vi "camera_acquisition_cooper.vi"(9 "Pixel Clock":dbl, 10 "Frame Rate":dbl) -> ()   [LabVIEW 2016]
uses:
  C:/Users/RegA/Box/bokor/cooper/32_bit/Library_X86/Thorlabs.TSI.ImageDataInterfaces.dll
  C:/Users/RegA/Box/bokor/cooper/32_bit/Library_X86/Thorlabs.TSI.TLCameraInterfaces.dll
  <vilib>/Analysis/NI_AALBase.lvlib
  C:/Users/RegA/Box/bokor/cooper/32_bit/Library_X86/Thorlabs.TSI.TLCamera.dll
  <vilib>/Analysis/baseanly.llb/A x Vector.vi
  <vilib>/Utility/file.llb/Write Delimited Spreadsheet (string).vi
  <vilib>/Utility/file.llb/Write Delimited Spreadsheet (DBL).vi
panel:
  in  "Subtract\nBackground":bool
  in  "Calibrate\nBackground":bool
  out "Background":u8[][](graph)
  in  "Stop Recording":bool
  out "Recording In\nProgress":bool
  in  "File Name (3):":string="GdFeCo202_"
  in  "Save at (3):":path=path "C:/Users/Bokor Group/Google Drive/MOKE_Microscopy/11_2016/Nov14"
  in  "Start Recording":bool
  out "Recording\nFrames":dbl
  out "Recording\nLength":dbl
  out "Scan in\nProgress":bool
  in  "Amplifier\nGPIB":refnum<visa-resource-name>="GPIB0::8::INSTR"
  in  "Enable Manual Control":bool
  in  "File Name (2):":string="GdFeCo202_"
  in  "Save at (2):":path=path "C:/Users/Bokor Group/Google Drive/MOKE_Microscopy/11_2016/Nov14"
  in  "Kepco\nGPIB":refnum<visa-resource-name>="GPIB0::8::INSTR"
  in  "Number\nOf Loops":dbl=1.0
  in  "Set I\nDelay":dbl=0.5
  in  "Stop\nScan":bool
  out "Hysteresis\nGraph":cluster{dbl[], dbl[]}(graph)={[0.0, 0.05, 0.1, 0.15000000000000002, 0.2, 0.25, 0.3, 0.0], [5.96051e-08, 8.56821e-08, 5.21543e-08, 2.98025e-08, 6.33304e-08, 7.0781e-08, 9.31327e-08, 1.00583e-07]}
  in  "Step (A)":dbl=0.05 format="%.5f"
  in  "-Imax (A)":dbl=-0.5
  in  "Imax (A)":dbl=0.5
  in  "Kepco Control Value":dbl(knob) min=-3.0 max=3.0 step=0.01 scale=-0.5..0.5 scale format="%#_3g"
  in  "Start\nScan":bool
  in  "Save\nScan":bool
  in  "File Name (1):":string="GdFeCo202_"
  in  "Save At (1):":path=path "C:/Users/Bokor Group/Google Drive/MOKE_Microscopy/11_2016/Nov14"
  in  "Take Pic":bool
  out "Pic Taken":u8[][](graph)
  in  "Exposure (ms)":u32=100
  in  "Intensity\nRange":cluster{dbl, dbl}(slide)={56.92307692307693, 40.0} scale=40.0..160.0
  out "Average":dbl=48.534001159667945
  out "Video":u8[][](graph)
  in  "Maximum\nIntensity":bool
  in  "stop":bool
  # "Save Pic"
  # "Save Video"
  # "Stop Button"
  # "Save Hysteresis Scan"
  # "Control Kepco"
  # "Background"
  # "A"
  # "Camera Image"
  # "Run Hysteresis Loop"
  # "Kepco GPIB"
  # "Unused"
  # "Amplifier GPIB"
  # "Unused"
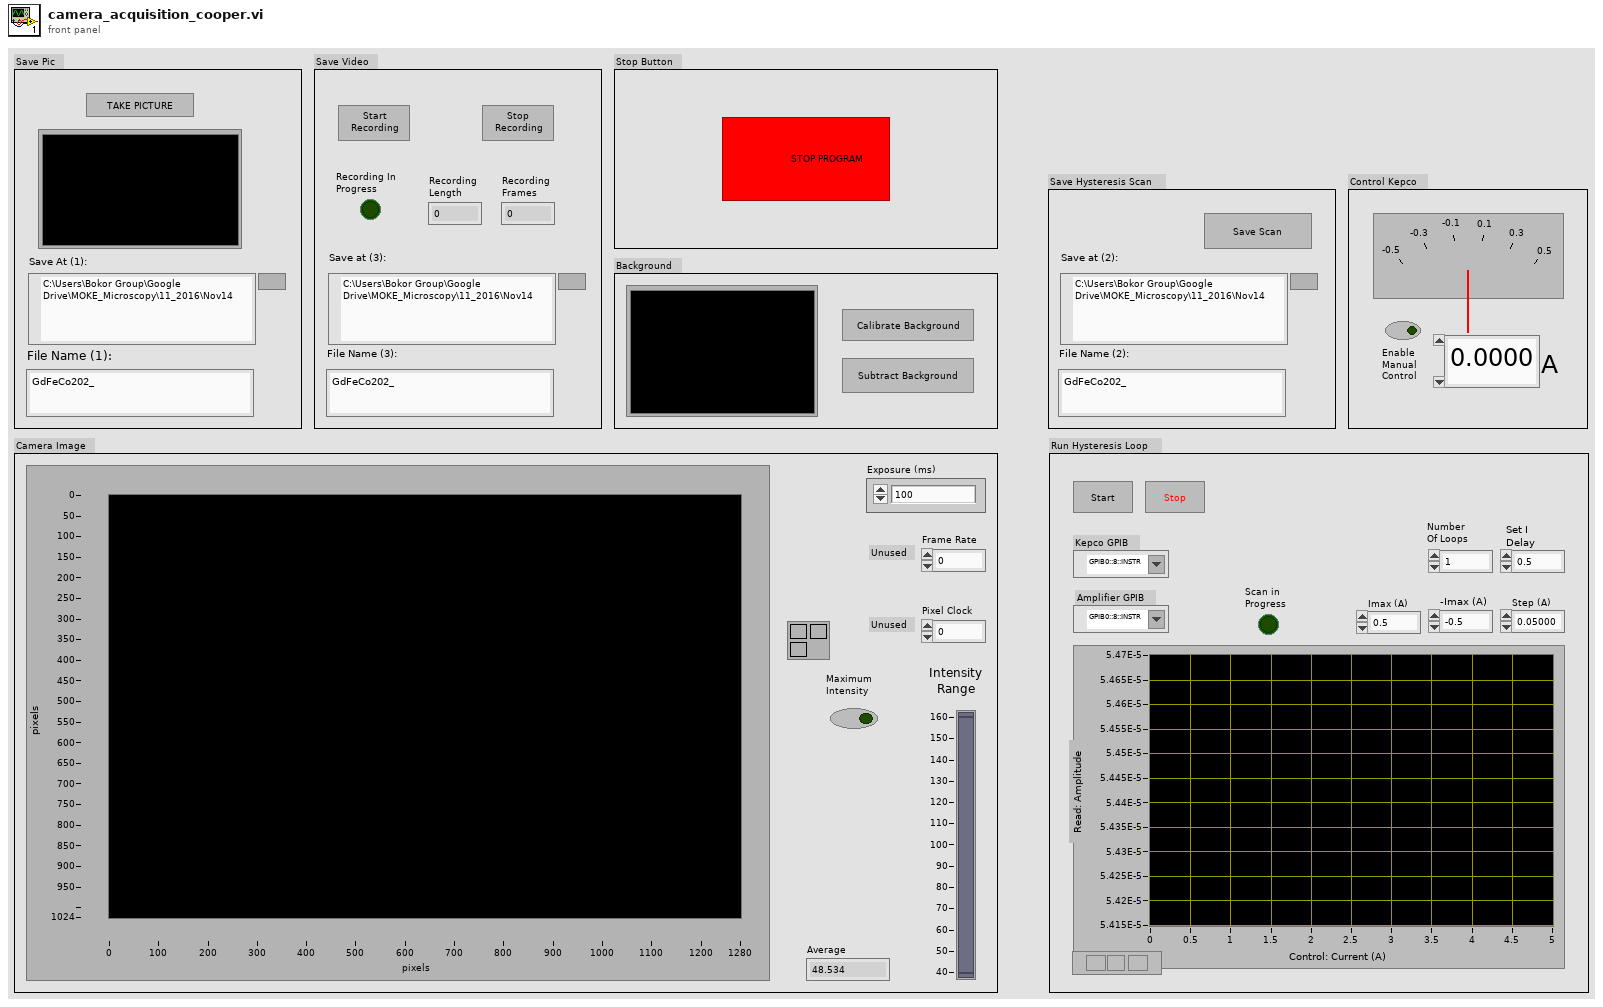
[diagram p1: front panel]
types:
  T1 = typedef "IMAQ Image.ctl" = refnum<image>
  T2 = typedef "AviRefnum.ctl" = refnum<k1>
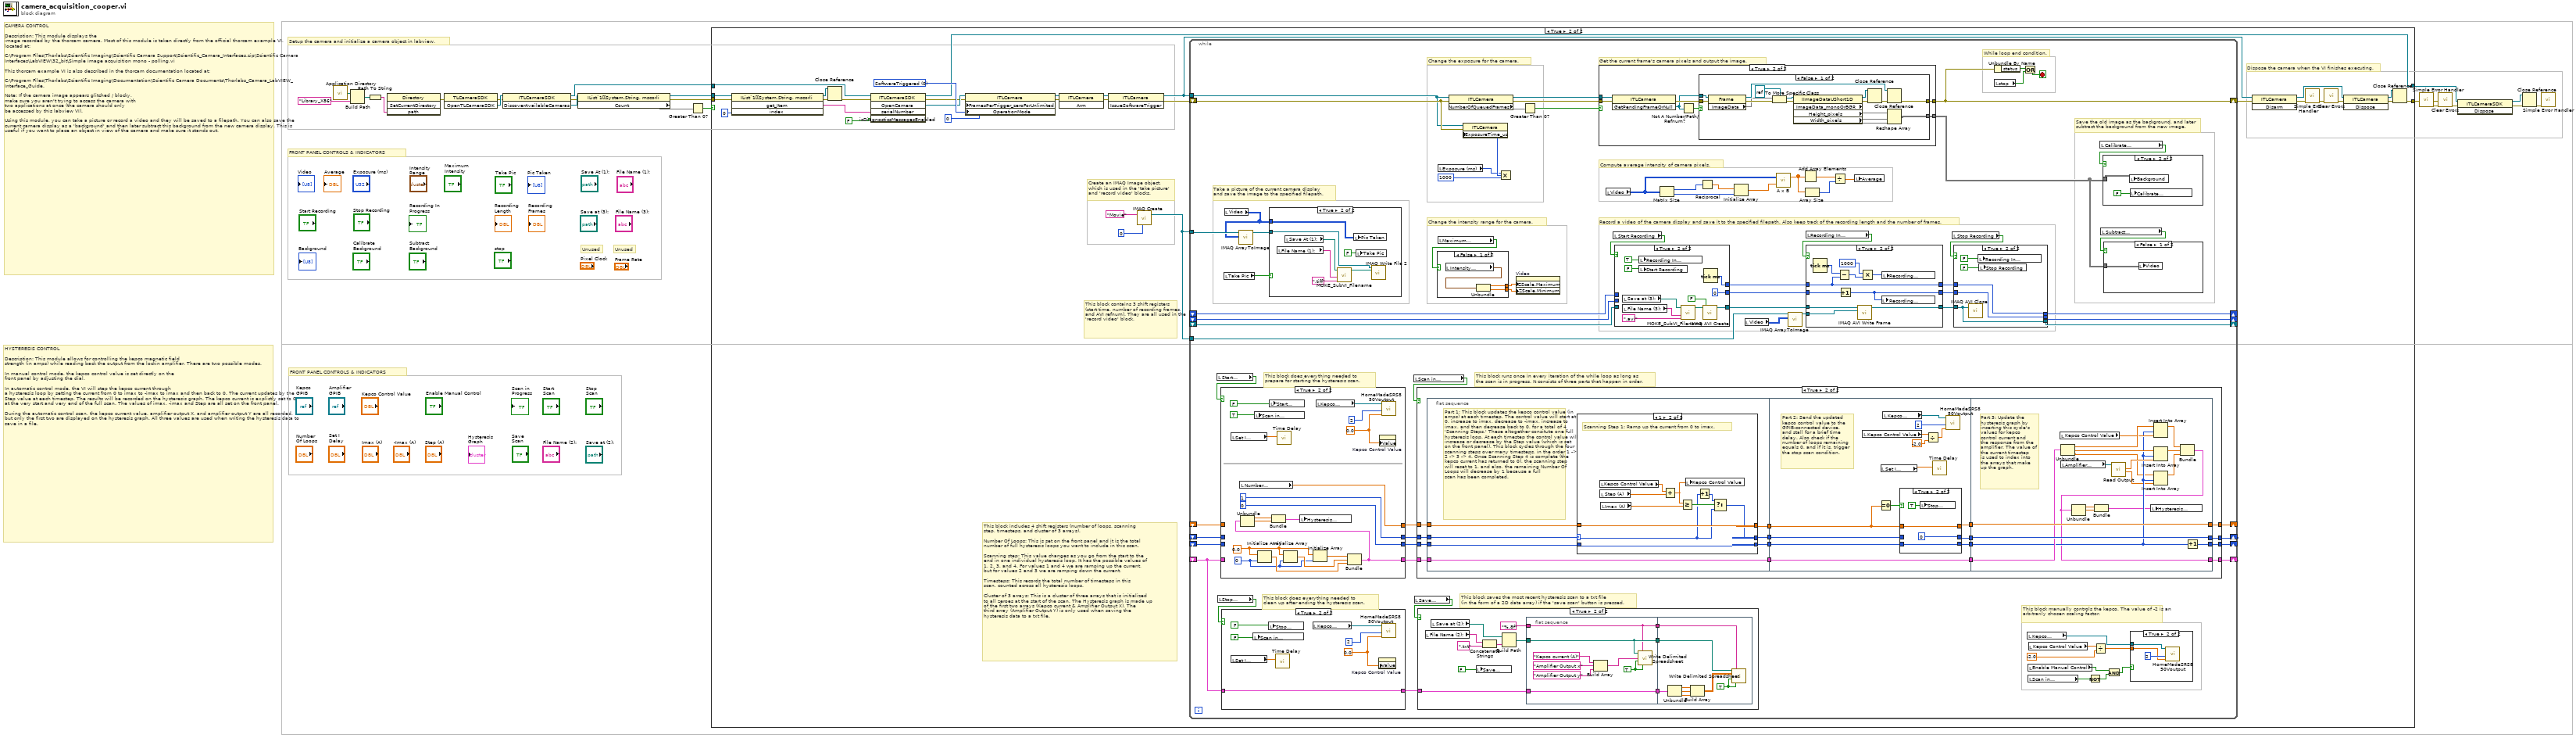
[diagram p0: block diagram]
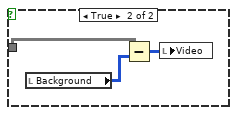
[diagram p3: hidden frame]
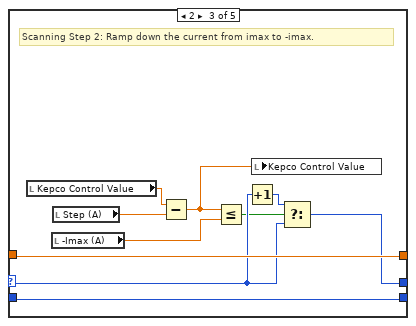
[diagram p12: hidden frame]
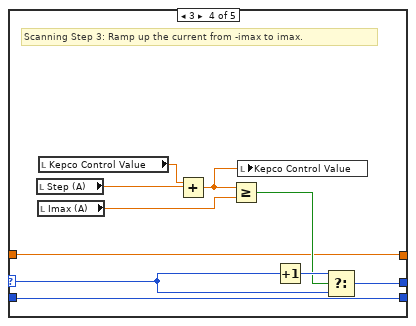
[diagram p13: hidden frame]
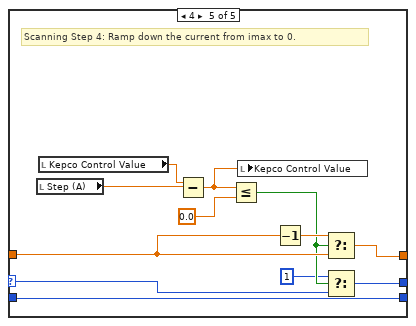
[diagram p14: hidden frame]
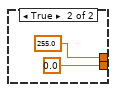
[diagram p19: hidden frame]
diagram:
  # "Unused"
  # "Unused"
  # "FRONT PANEL CONTROLS & INDICATORS"
  # "HYSTERESIS CONTROL\n\nDescription: This module allows for controlling the kepco magnetic field\nstrength (in amps) while reading back the output from the lockin amplifier. There are two possible modes. \n\nIn manual control mode, the kepco control value is set directly on the\nfront panel by adjusting the dial.\n\nIn automatic control mode, the VI will step the kepco current through\na hysteresis loop by setting the current from 0 to imax to -imax to imax and then back to 0. The current updates by the Step value at each timestep. The results will be recorded on the hysteresis graph. The kepco current is explictly set to 0 at the very start and very end of the full scan. The values of imax, -imax and Step are all set on the front panel.\n\nDuring the automatic control scan, the kepco current value, amplifier output X, and amplifier output Y are all recorded, but only the first two are displayed on the hysteresis graph. All three values are used when writing the hysteresis data to save in a file."
  # "CAMERA CONTROL\n\nDescription: This module displays the\nimage recorded by the thorcam camera. Most of this module is taken directly from the official thorcam example VI, located at:\n\nC:\\Program Files\\Thorlabs\\Scientific Imaging\\Scientific Camera Support\\Scientific_Camera_Interfaces.zip\\Scientific Camera Interfaces\\LabVIEW\\32_bit\\Simple image acquisition mono - polling.vi\n\nThis thorcam example VI is also described in the thorcam documentation located at:\n\nC:\\Program Files\\Thorlabs\\Scientific Imaging\\Documentation\\Scientific Camera Documents\\Thorlabs_Camera_LabVIEW_Interface_Guide.\n\nNote: If the camera image appears glitched / blocky,\nmake sure you aren't trying to access the camera with\ntwo applications at once (the camera should only\nbe accessed by this labview VI).\n\nUsing this module, you can take a picture or record a video and they will be saved to a filepath. You can also save the current camera display as a 'background' and then later subtract this background from the new camera display. This is useful if you want to place an object in view of the camera and make sure it stands out."
  # "Setup the camera and initialize a camera object in labview."
  # "FRONT PANEL CONTROLS & INDICATORS"
  n1 = call <vilib>:"Application Directory.vi"() -> ("Application Directory"=w14:path)
  n2 = Build Path(base path=w14, name or relative path="Library_X86") -> (appended path=w12:path)
  n3 = Path To String(path=w12) -> (string=w2:string)
  n4 = invoke class="Directory" method="SetCurrentDirectory"("path"=w2) -> (error out=w8:errorcluster)  [unwired: 3 in, 3 out]
  n5 = invoke class="TLCameraSDK" method="OpenTLCameraSDK"(error in=w8) -> (error out=w6:errorcluster, "OpenTLCameraSDK"=w7:refnum<k24>)  [unwired: 2 in, 1 out]
  n6 = invoke class="ITLCameraSDK" method="DiscoverAvailableCameras"(reference=w7, error in=w6) -> (reference out=w5:refnum<k24>, error out=w3:errorcluster, "DiscoverAvailableCameras"=w4:refnum<k24>)  [unwired: 1 in]
  n7 = property class="IList`1[[System.String, mscorli"(reference=w4, error in=w3) -> (reference out=w16:refnum<k24>, error out=w15:errorcluster, "Count"=w1)
  n8 = Greater Than 0?(x=w1) -> (x > 0?=w17:bool)
  n9 = case shown="True" w17 {
    tunnel: w5 -> [w22 w54]
    tunnel: w15 -> [w23 w48]
    tunnel: [w23 w50] -> w10
    tunnel: [w22 w26] -> w21
    tunnel: w16 -> [_ w49]
    frame False {
    }
    frame True {
      w41 = 0 items=["SoftwareTriggered", "HardwareTriggered", "Bulb", "Reserved1", "Reserved2"] ("OperationMode")
      # "This block contains 3 shift registers (start time, number of recording frames, and AVI refnum). They are all used in the 'record video' block."
      # "Create an IMAQ Image object,\nwhich is used in the 'take picture'\nand 'record video' blocks."
      # "Dispose the camera when the VI finishes executing."
      # "This block includes 4 shift registers (number of loops, scanning\nstep, timesteps, and cluster of 3 arrays).\n\nNumber Of Loops: This is set on the front panel and it is the total\nnumber of full hysteresis loops you want to include in this scan.\n\nScanning step: This value changes as you go from the start to the\nend in one individual hysteresis loop. It has the possible values of\n1, 2, 3, and 4. For values 1 and 4 we are ramping up the current,\nbut for values 2 and 3 we are ramping down the current.\n\nTimesteps: This records the total number of timesteps in this\nscan, counted across all hysteresis loops.\n\nCluster of 3 arrays: This is a cluster of three arrays that is initialized\nto all zeroes at the start of the scan. The Hysteresis graph is made up \nof the first two arrays (Kepco current & Amplifier Output X). The\nthird array (Amplifier Output Y) is only used when saving the \nhysteresis data to a txt file."
      n10 = invoke class="IList`1[[System.String, mscorli" method="get_Item"(reference=w49, error in=w48, "index"=0) -> (reference out=w47:refnum<k24>, error out=w46:errorcluster, "get_Item"=w44:string)  [unwired: 1 in, 1 out]
      n11 = Close Reference(reference=w47, error in (no error)=w46) -> (error out=w45:errorcluster)
      n12 = invoke class="ITLCameraSDK" method="OpenCamera"(reference=w54, error in=w45, "serialNumber"=w44, "isDiagnosticsMessagesEnabled"=FALSE) -> (reference out=w26:refnum<k24>, error out=w33:errorcluster, "OpenCamera"=w34:refnum<k24>)  [unwired: 1 in, 2 out]
      n13 = property class="ITLCamera"(reference=w34, error in=w33, "FramesPerTrigger_zeroForUnlimited"=u32 0 ("FramesPerTriggerOrZeroForUnlimited"), "OperationMode"=w41) -> (reference out=w36:refnum<k24>, error out=w35:errorcluster)
      n14 = invoke class="ITLCamera" method="Arm"(reference=w36, error in=w35) -> (reference out=w43:refnum<k24>, error out=w42:errorcluster)  [unwired: 1 in, 1 out]
      n15 = invoke class="ITLCamera" method="IssueSoftwareTrigger"(reference=w43, error in=w42) -> (reference out=w27:refnum<k24>, error out=w24:errorcluster)  [unwired: 1 in, 1 out]
      n16 = call "IMAQ Create"("Image Name"="Movie", "Image Type"=0) -> ("New Image"=w25:T1)  [unwired: 3 in, 1 out]
      n17 = while {
        tunnel: w27 -> [w110]
        shift-right: [w84] -> w40
        shift-left: w24 -> [w118]
        tunnel: w25 -> [w117]
        shift-right: [w98] -> _
        shift-left: _ -> [w66]
        shift-right: [w97] -> _
        shift-left: _ -> [w67]
        shift-right: [w99] -> _
        shift-left: _ -> [w65]
        shift-right: [w92] -> _
        shift-left: _ -> [w96]
        shift-right: [w86] -> _
        shift-left: _ -> [w89]
        shift-right: [w75] -> _
        shift-left: _ -> [w85]
        tunnel: w25 -> [w80]
        shift-right: [w64] -> _
        shift-left: _ -> [w61]
        stop <- w129 stop-if-true
        # "Save the old image as the background, and later\nsubtract the background from the new image."
        # "Take a picture of the current camera display\nand save the image to the specified filepath."
        # "Record a video of the camera display and save it to the specified filepath. Also keep track of the recording length and the number of frames."
        # "This block saves the most recent hysteresis scan to a txt file \n(in the form of a 2D data array) if the 'save scan' button is pressed."
        # "This block runs once in every iteration of the while loop as long as\nthe scan is in progress. It consists of three parts that happen in order."
        # "While loop end condition."
        # "This block does everything needed to\nclean up after ending the hysteresis scan."
        # "This block does everything needed to\nprepare for starting the hysteresis scan."
        # "This block manually controls the kepco. The value of -2 is an arbitrarily chosen scaling factor."
        # "Get the current frame's camera pixels and output the image."
        # "Change the intensity range for the camera."
        # "Compute average intensity of camera pixels."
        # "Change the exposure for the camera."
        n18 = local read "Start\nScan"() -> (w73:bool)
        n19 = local read "Stop\nScan"() -> (w63:bool)
        n20 = case shown="True" w73 {
          tunnel: [w320 w323] -> w71
          tunnel: w61 -> [w320 _]
          tunnel: [w319 w327] -> w70
          tunnel: [w318 1] -> w69
          tunnel: [w317 0] -> w68
          tunnel: w67 -> [w319 _]
          tunnel: w66 -> [w318 _]
          tunnel: w65 -> [w317 _]
          frame False {
          }
          frame True {
            w329 = 0.0
            w328 = 0
            w335 = 0.0
            n21 = local read "Set I\nDelay"() -> (w333:dbl)
            n22 = local read "Number\nOf Loops"() -> (w327:dbl)
            n23 = local write "Scan in\nProgress"(TRUE) -> ()
            n24 = Initialize Array(w329, w328) -> (w332:dbl[])
            n25 = local write "Start\nScan"(FALSE) -> ()
            n26 = call "Time Delay"("Delay Time (s)"=w333) -> ()  [unwired: 10 in, 1 out]
            n27 = Initialize Array(w329, w328) -> (w331:dbl[])
            n28 = Initialize Array(w329, w328) -> (w330:dbl[])
            n29 = local read "Kepco\nGPIB"() -> (w334:refnum<visa-resource-name>)
            n30 = Bundle(w330, w331, w332) -> (w323:cluster{dbl[], dbl[], dbl[]})  [unwired: 1 in]
            n31 = Unbundle(w323) -> (w322:dbl[], w321:dbl[])  [unwired: 1 out]
            n32 = Bundle(w322, w321) -> (w324:cluster{dbl[], dbl[]})  [unwired: 1 in]
            n33 = local write "Hysteresis\nGraph"(w324) -> ()
            n34 = property on="Kepco Control Value" class="Knob (strict)"("Value"=w335) -> ()  [unwired: 2 in, 2 out]
            n35 = call "HomeMadeSRS850Voutput.vi"("V output"=w335, "Aux. Channel"=2, "VISA resource name"=w334) -> ()  [unwired: 7 in, 2 out]
          }
        }
        n36 = case shown="True" w63 {
          tunnel: w61 -> [w197 w198]
          tunnel: [w197 w198] -> w62
          frame False {
          }
          frame True {
            w202 = 0.0
            n37 = local read "Set I\nDelay"() -> (w199:dbl)
            n38 = local write "Scan in\nProgress"(FALSE) -> ()
            n39 = local write "Stop\nScan"(FALSE) -> ()
            n40 = call "Time Delay"("Delay Time (s)"=w199) -> ()  [unwired: 10 in, 1 out]
            n41 = local read "Kepco\nGPIB"() -> (w200:refnum<visa-resource-name>)
            n42 = property on="Kepco Control Value" class="Knob (strict)"("Value"=w202) -> ()  [unwired: 2 in, 2 out]
            n43 = call "HomeMadeSRS850Voutput.vi"("V output"=w202, "Aux. Channel"=2, "VISA resource name"=w200) -> ()  [unwired: 7 in, 2 out]
          }
        }
        n44 = local read "Take Pic"() -> (w108:bool)
        n45 = local read "Video"() -> (w109:u8[][])
        n46 = call "IMAQ ArrayToImage"("Image Pixels (U8)"=w109, "Image"=w117) -> ("Image Out"=w116:T1)  [unwired: 8 in, 1 out]
        n47 = case shown="True" w108 {
          tunnel: w116 -> [_ w345]
          tunnel: w109 -> [_ w343]
          frame False {
          }
          frame True {
            n48 = local read "File Name (1):"() -> (w342:string)
            n49 = local read "Save At (1):"() -> (w346:path)
            n50 = call "MOKE_SubVI_Filename.vi"("extension"=".tiff" ("pattern"), "File Name:"=w342, "Save at:"=w346) -> ("FULL Path"=w348:path)  [unwired: 6 in, 2 out]
            n51 = local write "Pic Taken"(w343) -> ()
            n52 = local write "Take Pic"(FALSE) -> ()
            n53 = call-poly "IMAQ Write File 2"("File Path"=w348, "Image"=w345) -> ()  [unwired: 8 in, 2 out]
          }
        }
        n54 = local read "Scan in\nProgress"() -> (w72:bool)
        n55 = local read "Save\nScan"() -> (w60:bool)
        n56 = case shown="True" w72 {
          tunnel: w70 -> [w208 w223]
          tunnel: w69 -> [w207 w224]
          tunnel: [w207 w222] -> w98
          tunnel: [w208 w221] -> w97
          tunnel: w68 -> [w206 w215]
          tunnel: [w206 w213] -> w99
          tunnel: w71 -> [w205 w212]
          tunnel: [w205 w209] -> w64
          frame False {
          }
          frame True {
            n57 = flat-sequence {
              tunnel: w224 -> [w231]
              tunnel: w223 -> [w230]
              tunnel: [w229] -> w220
              tunnel: [w228] -> w219
              tunnel: [w227] -> w216
              tunnel: w215 -> [w226]
              tunnel: w212 -> [w225]
              tunnel: [w225] -> w211
              tunnel: w220 -> [w289]
              tunnel: w219 -> [w288]
              tunnel: [w286] -> w218
              tunnel: [w287] -> w217
              tunnel: w216 -> [w283]
              tunnel: [w282] -> w214
              tunnel: w211 -> [w277]
              tunnel: [w277] -> w210
              tunnel: [w315] -> w221
              tunnel: [w316] -> w222
              tunnel: w218 -> [w316]
              tunnel: w217 -> [w315]
              tunnel: w214 -> [w304]
              tunnel: [w314] -> w213
              tunnel: w210 -> [w306]
              tunnel: [w301] -> w209
              frame #0 {
                # "Part 1: This block updates the kepco control value (in amps) at each timestep. The control value will start at 0, increase to imax, decrease to -imax, increase to imax, and then decrease back to 0, for a total of 4 'Scanning Steps.' These altogether consitute one full hysteresis loop. At each timestep the control value will increase or decrease by the Step value (which is set on the front panel). This block cycles through the four scanning steps over many timesteps, in the order 1 -> 2 -> 3 -> 4. Once Scanning Step 4 is complete (the kepco current has returned to 0), the scanning step will reset to 1, and also, the remaining Number Of Loops will decrease by 1 because a full\nscan has been completed."
                n58 = case shown="1" w231 {
                  selector: w231 -> [w233 w235 w252 w255 w266]
                  tunnel: [w233 w237 w251 w261 w272] -> w229
                  tunnel: [w234 w244 w254 w256 w270] -> w228
                  tunnel: w230 -> [w234 w244 w254 w256 w269]
                  tunnel: [w232 w236 w246 w260 w271] -> w227
                  tunnel: w226 -> [w232 w236 w246 w260 w271]
                  frame 0, Default {
                  }
                  frame 1 {
                    # "Scanning Step 1: Ramp up the current from 0 to imax."
                    n59 = local read "Kepco Control Value"() -> (w243:dbl)
                    n60 = local read "Step (A)"() -> (w242:dbl)
                    n61 = local read "Imax (A)"() -> (w240:dbl)
                    n62 = Add(x=w243, y=w242) -> (x+y=w241:dbl)
                    n63 = Greater Or Equal?(x=w241, y=w240) -> (x >= y?=w239:bool)
                    n64 = local write "Kepco Control Value"(w241) -> ()
                    n65 = Increment(x=w235) -> (x+1=w238:i32)
                    n66 = Select(t=w238, s=w239, f=w235) -> (s? t:f=w237:i32)
                  }
                  frame 2 {
                    # "Scanning Step 2: Ramp down the current from imax to -imax."
                    n67 = local read "Kepco Control Value"() -> (w250:dbl)
                    n68 = local read "-Imax (A)"() -> (w245:dbl)
                    n69 = local read "Step (A)"() -> (w249:dbl)
                    n70 = Subtract(x=w250, y=w249) -> (x-y=w248:dbl)
                    n71 = Less Or Equal?(x=w248, y=w245) -> (x <= y?=w247:bool)
                    n72 = Increment(x=w252) -> (x+1=w253:i32)
                    n73 = local write "Kepco Control Value"(w248) -> ()
                    n74 = Select(t=w253, s=w247, f=w252) -> (s? t:f=w251:i32)
                  }
                  frame 3 {
                    # "Scanning Step 3: Ramp up the current from -imax to imax."
                    n75 = local read "Step (A)"() -> (w263:dbl)
                    n76 = local read "Imax (A)"() -> (w257:dbl)
                    n77 = local read "Kepco Control Value"() -> (w264:dbl)
                    n78 = Add(x=w264, y=w263) -> (x+y=w262:dbl)
                    n79 = Greater Or Equal?(x=w262, y=w257) -> (x >= y?=w258:bool)
                    n80 = local write "Kepco Control Value"(w262) -> ()
                    n81 = Increment(x=w255) -> (x+1=w259:i32)
                    n82 = Select(t=w259, s=w258, f=w255) -> (s? t:f=w261:i32)
                  }
                  frame 4 {
                    # "Scanning Step 4: Ramp down the current from imax to 0."
                    n83 = local read "Step (A)"() -> (w275:dbl)
                    n84 = local read "Kepco Control Value"() -> (w276:dbl)
                    n85 = Subtract(x=w276, y=w275) -> (x-y=w274:dbl)
                    n86 = Less Or Equal?(x=w274, y=0.0) -> (x <= y?=w268:bool)
                    n87 = local write "Kepco Control Value"(w274) -> ()
                    n88 = Decrement(x=w269) -> (x-1=w273:dbl)
                    n89 = Select(t=w273, s=w268, f=w269) -> (s? t:f=w270:dbl)
                    n90 = Select(t=1, s=w268, f=w266) -> (s? t:f=w272:i32)
                  }
                }
              }
              frame #1 {
                # "Part 2: Send the updated \nkepco control value to the\nGPIB-connected device,\nand stall for a brief time \ndelay. Also check if the\nnumber of loops remaining\nequals 0, and if it is, trigger\nthe stop scan condition."
                n91 = local read "Kepco Control Value"() -> (w281:dbl)
                n92 = Equal To 0?(x=w288) -> (x = 0?=w290:bool)
                n93 = local read "Set I\nDelay"() -> (w284:dbl)
                n94 = local read "Kepco\nGPIB"() -> (w279:refnum<visa-resource-name>)
                n95 = case shown="True" w290 {
                  tunnel: [w293 0] -> w286
                  tunnel: w289 -> [w293 _]
                  tunnel: w288 -> [w292 w296]
                  tunnel: [w292 w296] -> w287
                  tunnel: [w291 w295] -> w282
                  tunnel: w283 -> [w291 w295]
                  frame False {
                  }
                  frame True {
                    n96 = local write "Stop\nScan"(TRUE) -> ()
                  }
                }
                n97 = Divide(x=w281, y=-2.0) -> (x/y=w285:dbl)
                n98 = call "Time Delay"("Delay Time (s)"=w284) -> ()  [unwired: 10 in, 1 out]
                n99 = call "HomeMadeSRS850Voutput.vi"("V output"=w285, "Aux. Channel"=2, "VISA resource name"=w279) -> ()  [unwired: 7 in, 2 out]
              }
              frame #2 {
                # "Part 3: Update the\nhysteresis graph by\ninserting this cycle's\nvalues for kepco\ncontrol current and \nthe response from the\namplifier. The value of\nthe current timestep\nis used to index into\nthe arrays that make\nup the graph."
                n100 = local read "Kepco Control Value"() -> (w310:dbl)
                n101 = Unbundle(w306) -> (w312:dbl[], w311:dbl[], w303:dbl[])
                n102 = local read "Amplifier\nGPIB"() -> (w313:refnum<visa-resource-name>)
                n103 = call "Read Output.vi"("VISA resource name"=w313) -> ("Y"=w302:dbl, "X"=w309:dbl)  [unwired: 5 in, 4 out]
                n104 = Insert Into Array(array=w312, index=w304, new element=w310) -> (w308:dbl[])
                n105 = Insert Into Array(array=w311, index=w304, new element=w309) -> (w307:dbl[])
                n106 = Insert Into Array(array=w303, index=w304, new element=w302) -> (w305:dbl[])
                n107 = Bundle(w308, w307, w305) -> (w301:cluster{dbl[], dbl[], dbl[]})  [unwired: 1 in]
                n108 = Unbundle(w301) -> (w300:dbl[], w299:dbl[])  [unwired: 1 out]
                n109 = Bundle(w300, w299) -> (w298:cluster{dbl[], dbl[]})  [unwired: 1 in]
                n110 = local write "Hysteresis\nGraph"(w298) -> ()
                n111 = Increment(x=w304) -> (x+1=w314:i32)
              }
            }
          }
        }
        n112 = case shown="True" w60 {
          tunnel: w62 -> [_ w180]
          frame False {
          }
          frame True {
            n113 = local read "File Name (2):"() -> (w177:string)
            n114 = local read "Save at (2):"() -> (w178:path)
            n115 = local write "Save\nScan"(FALSE) -> ()
            n116 = Concatenate Strings(w177, ".txt" ("string")) -> (w176:string)
            n117 = Build Path(base path=w178, name or relative path=w176) -> (appended path=w174:path)
            n118 = flat-sequence {
              tunnel: w174 -> [w187]
              tunnel: w180 -> [w188]
              tunnel: [w188] -> w173
              tunnel: "%.8f" ("format (%.3f)") -> [w186]
              tunnel: [w187] -> w171
              tunnel: [w186] -> w170
              tunnel: w173 -> [w194]
              tunnel: w171 -> [w190]
              tunnel: w170 -> [w189]
              frame #0 {
                w185 = TRUE
                n119 = Build Array("Kepco current (A)", "Amplifier Output x", "Amplifier Output y") -> (w181:string[])
                n120 = call-poly <vilib>:"Write Delimited Spreadsheet.vi"("file path (dialog if empty)"=w187, "format (%s)"=w186, "1D data"=w181, "append to file? (new file:F)"=w185, "transpose? (no:F)"=w185) -> ()  [unwired: 9 in, 2 out]
              }
              frame #1 {
                w195 = TRUE ("Take Pic")
                n121 = Unbundle(w194) -> (w193:dbl[], w192:dbl[], w191:dbl[])
                n122 = Build Array(w193, w192, w191) -> (w196:dbl[][])
                n123 = call-poly <vilib>:"Write Delimited Spreadsheet.vi"("file path (dialog if empty)"=w190, "format (%.3f)"=w189, "2D data"=w196, "append to file? (new file:F)"=w195, "transpose? (no:F)"=w195) -> ()  [unwired: 9 in, 2 out]
              }
            }
          }
        }
        n124 = local read "Exposure (ms)"() -> (w77:u32)
        n125 = local read "Maximum\nIntensity"() -> (w83:bool)
        n126 = case shown="False" w83 {
          tunnel: [w350 255.0] -> w120
          tunnel: [w349 0.0] -> w119
          frame False {
            n127 = local read "Intensity\nRange"() -> (w351:cluster{dbl, dbl})
            n128 = Unbundle(w351) -> (w350:dbl, w349:dbl)
          }
          frame True {
          }
        }
        n129 = property class="ITLCamera"(reference=w110, error in=w118) -> (reference out=w113:refnum<k24>, error out=w112:errorcluster, "NumberOfQueuedFrames"=w111)
        n130 = Multiply(x=w77, y=1000) -> (x*y=w79:u32)
        n131 = property class="ITLCamera"(reference=w110, error in=w118, "ExposureTime_us"=w79) -> ()  [unwired: 2 out]
        n132 = property on="Video" class="IntGraph (strict)"("ZScale.Maximum"=w120, "ZScale.Minimum"=w119) -> ()  [unwired: 2 in, 2 out]
        n133 = Greater Than 0?(x=w111) -> (x > 0?=w114:bool)
        n134 = case shown="True" w114 {
          tunnel: w112 -> [w354 w360]
          tunnel: w113 -> [_ w361]
          tunnel: [w354 w356] -> w84
          tunnel: [_ w355] -> w57
          frame False {
          }
          frame True {
            n135 = invoke class="ITLCamera" method="GetPendingFrameOrNull"(reference=w361, error in=w360) -> (error out=w357:errorcluster, "GetPendingFrameOrNull"=w358:refnum<k24>)  [unwired: 1 in, 1 out]
            n136 = Not A Number/Path/Refnum?(number/path/refnum=w358) -> (NaN/Path/Refnum?=w359:bool)
            n137 = case shown="False" w359 {
              tunnel: w358 -> [w368 _]
              tunnel: w357 -> [w376 w378]
              tunnel: [w371 w378] -> w356
              tunnel: [w362 _] -> w355
              frame False {
                n138 = property class="Frame"(reference=w368, error in=w376) -> (reference out=w373:refnum<k24>, error out=w366:errorcluster, "ImageData"=w367)
                n139 = To More Specific Class(target class=refnum<k24> refnum, reference=w367, error in=w366) -> (specific class reference=w364:refnum<k24>, error out=w365:errorcluster)
                n140 = property class="IImageDataUShort1D"(reference=w364, error in=w365) -> (reference out=w374:refnum<k24>, error out=w375:errorcluster, "ImageData_monoOrBGR"=w377, "Height_pixels"=w369, "Width_pixels"=w370)
                n141 = Close Reference(reference=w374, error in (no error)=w375) -> (error out=w372:errorcluster)
                n142 = Close Reference(reference=w373, error in (no error)=w372) -> (error out=w371:errorcluster)
                n143 = Reshape Array(w377, w369, w370) -> (w362:void[][])
              }
              frame True {
              }
            }
          }
        }
        n144 = local read "Video"() -> (w55:u8[][])
        n145 = local read "Start Recording"() -> (w94:bool)
        n146 = case shown="True" w94 {
          tunnel: [w159 w166] -> w95
          tunnel: w96 -> [w159 _]
          tunnel: w89 -> [w158 _]
          tunnel: [w158 0] -> w88
          tunnel: w85 -> [w157 _]
          tunnel: [w157 w161] -> w76
          frame False {
          }
          frame True {
            n147 = local read "Save at (3):"() -> (w163:path)
            n148 = local read "File Name (3):"() -> (w164:string)
            n149 = local write "Recording In\nProgress"(TRUE) -> ()
            n150 = local write "Start Recording"(FALSE) -> ()
            n151 = call "MOKE_SubVI_Filename.vi"("extension"=".avi", "File Name:"=w164, "Save at:"=w163) -> ("FULL Path"=w168:path)  [unwired: 6 in, 2 out]
            n152 = call "IMAQ AVI Create"("Has Data"=FALSE, "AVI Path"=w168) -> ("Avi Refnum"=w166:T2)  [unwired: 8 in, 1 out]
            n153 = Tick Count (ms)() -> (millisecond timer value=w161:u32)
          }
        }
        n154 = Matrix Size(0:w55) -> (1:w122:i32, 2:w128:i32)
        n155 = Reciprocal(x=w122) -> (1/x=w123:dbl)
        n156 = Initialize Array(w123, w128) -> (w124:dbl[])
        n157 = local read "Video"() -> (w81:u8[][])
        n158 = call-poly <vilib>:"A x B.vi"("Vector"=w124, "A"=w55) -> ("A x Vector"=w127:dbl[])  [unwired: 1 out]
        n159 = call "IMAQ ArrayToImage"("Image Pixels (U8)"=w81, "Image"=w80) -> ("Image Out"=w82:T1)  [unwired: 8 in, 1 out]
        n160 = Add Array Elements(numeric array=w127) -> (sum=w126:dbl)
        n161 = Array Size(array=w127) -> (size(s)=w125:i32)
        n162 = local read "Recording In\nProgress"() -> (w90:bool)
        n163 = case shown="True" w90 {
          tunnel: w95 -> [w146 w156]
          tunnel: [w146 w147] -> w93
          tunnel: w88 -> [w145 w155]
          tunnel: [w145 w148] -> w87
          tunnel: w82 -> [_ w154]
          tunnel: w76 -> [w144 w149]
          tunnel: [w144 w149] -> w74
          frame False {
          }
          frame True {
            n164 = Tick Count (ms)() -> (millisecond timer value=w153:u32)
            n165 = Subtract(x=w153, y=w149) -> (x-y=w152:u32)
            n166 = Increment(x=w155) -> (x+1=w148:i32)
            n167 = call "IMAQ AVI Write Frame"("Image"=w154, "Avi Refnum"=w156) -> ("Avi Refnum (duplicate)"=w147:T2)  [unwired: 8 in, 1 out]
            n168 = Multiply(x=1000, y=w152) -> (x*y=w150:u32)
            n169 = local write "Recording\nFrames"(w148) -> ()
            n170 = local write "Recording\nLength"(w150) -> ()
          }
        }
        n171 = Divide(x=w126, y=w125) -> (x/y=w121:dbl)
        n172 = local write "Average"(w121) -> ()
        n173 = local read "Stop Recording"() -> (w91:bool)
        n174 = case shown="True" w91 {
          tunnel: w93 -> [w138 w142]
          tunnel: [w138 w142] -> w92
          tunnel: w87 -> [w137 w141]
          tunnel: [w137 w141] -> w86
          tunnel: [w136 w139] -> w75
          tunnel: w74 -> [w136 w139]
          frame False {
          }
          frame True {
            n175 = call "IMAQ AVI Close"("Avi Refnum"=w142) -> ()  [unwired: 10 in, 1 out]
            n176 = local write "Recording In\nProgress"(FALSE) -> ()
            n177 = local write "Stop Recording"(FALSE) -> ()
          }
        }
        n178 = Unbundle By Name(w84) -> ("status"=w115:bool)
        n179 = local read "stop"() -> (w56:bool)
        n180 = Or(x=w115, y=w56) -> (x .or. y?=w129:bool)
        n181 = local read "Kepco\nGPIB"() -> (w105:refnum<visa-resource-name>)
        n182 = local read "Enable Manual Control"() -> (w102:bool)
        n183 = local read "Scan in\nProgress"() -> (w103:bool)
        n184 = local read "Kepco Control Value"() -> (w107:dbl)
        n185 = Not(x=w103) -> (.not. x?=w101:bool)
        n186 = Divide(x=w107, y=-2.0) -> (x/y=w106:dbl)
        n187 = local read "Calibrate\nBackground"() -> (w59:bool)
        n188 = local read "Subtract\nBackground"() -> (w58:bool)
        n189 = case shown="True" w59 {
          tunnel: w57 -> [_ w135]
          frame False {
          }
          frame True {
            n190 = local write "Background"(w135) -> ()
            n191 = local write "Calibrate\nBackground"(FALSE) -> ()
          }
        }
        n192 = case shown="False" w58 {
          tunnel: w57 -> [w130 w133]
          frame False {
            n193 = local write "Video"(w130) -> ()
          }
          frame True {
            n194 = local read "Background"() -> (w132:u8[][])
            n195 = Subtract(x=w133, y=w132) -> (x-y=w131:u8[][])
            n196 = local write "Video"(w131) -> ()
          }
        }
        n197 = And(x=w102, y=w101) -> (x .and. y?=w100:bool)
        n198 = case shown="True" w100 {
          tunnel: w106 -> [_ w340]
          tunnel: w105 -> [_ w339]
          frame False {
          }
          frame True {
            n199 = call "HomeMadeSRS850Voutput.vi"("V output"=w340, "Aux. Channel"=u16 2 ("input 1"), "VISA resource name"=w339) -> ()  [unwired: 7 in, 2 out]
          }
        }
      }
      n200 = invoke class="ITLCamera" method="Disarm"(reference=w27, error in=w40) -> (reference out=w53:refnum<k24>, error out=w39:errorcluster)  [unwired: 1 in, 1 out]
      n201 = call <vilib>:"Simple Error Handler.vi"("error in (no error)"=w39) -> ("error out"=w38:errorcluster)  [unwired: 4 in, 4 out]
      n202 = call <vilib>:"Clear Errors.vi"("error in (no error)"=w38) -> ("error out"=w37:errorcluster)  [unwired: 5 in, 1 out]
      n203 = invoke class="ITLCamera" method="Dispose"(reference=w53, error in=w37) -> (reference out=w51:refnum<k24>, error out=w52:errorcluster)  [unwired: 1 in, 1 out]
      n204 = Close Reference(reference=w51, error in (no error)=w52) -> (error out=w50:errorcluster)
    }
  }
  n205 = call <vilib>:"Simple Error Handler.vi"("error in (no error)"=w10) -> ("error out"=w11:errorcluster)  [unwired: 4 in, 4 out]
  n206 = call <vilib>:"Clear Errors.vi"("error in (no error)"=w11) -> ("error out"=w9:errorcluster)  [unwired: 5 in, 1 out]
  n207 = invoke class="ITLCameraSDK" method="Dispose"(reference=w21, error in=w9) -> (reference out=w20:refnum<k24>, error out=w19:errorcluster)  [unwired: 1 in, 1 out]
  n208 = Close Reference(reference=w20, error in (no error)=w19) -> (error out=w18:errorcluster)
  n209 = call <vilib>:"Simple Error Handler.vi"("error in (no error)"=w18) -> ()  [unwired: 4 in, 5 out]
